vi "FormatTime.vi"(3 "secondNum":i32) -> (0 "secondText":string, 1 "timeText":string)   [LabVIEW 2015]
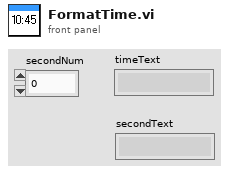
[diagram p1: front panel]
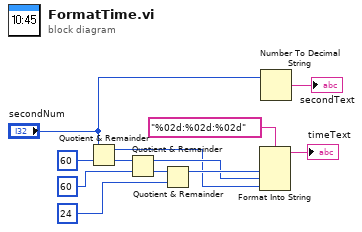
[diagram p0: block diagram]
diagram:
  n1 = Quotient & Remainder(x="secondNum", y=u32 60) -> (x-y*floor(x/y)=w4:u32, floor(x/y)=w10:u32)
  n2 = Quotient & Remainder(x=w10, y=u32 60) -> (x-y*floor(x/y)=w5:u32, floor(x/y)=w9:u32)
  n3 = Quotient & Remainder(x=w9, y=u32 24) -> (x-y*floor(x/y)=w6:u32)  [unwired: 1 out]
  n4 = Format Into String(format string="%02d:%02d:%02d", w6, w5, w4) -> (resulting string=→"timeText":string)  [unwired: 2 in, 1 out]
  n5 = Number To Decimal String(number="secondNum") -> (decimal integer string=→"secondText":string)  [unwired: 1 in]
